vi "Drive Output Ramp.vi"(7 "reinitialize?":bool, 10 "Right":dbl, 11 "Left":dbl) -> (2 "Right Output":dbl, 3 "Left Output":dbl)   [LabVIEW 2013]
uses:
  <vilib>/addons/control/pid/pid.llb/PID Output Rate Limiter (DBL Array).vi
  <vilib>/addons/control/pid/NI_PID_pid.lvlib
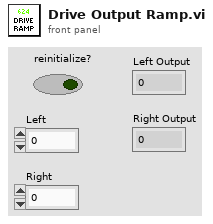
[diagram p1: front panel]
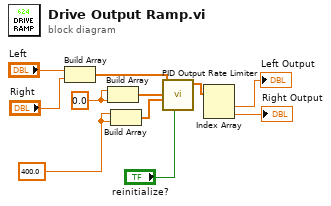
[diagram p0: block diagram]
diagram:
  w7 = 400.0 ("output rate (EGU/min)")
  w5 = 0.0 ("initial output")
  n1 = Build Array("Left", "Right") -> (w2:dbl[])
  n2 = Build Array(w5, w5) -> (w6:dbl[])
  n3 = Build Array(w7, w7) -> (w8:dbl[])
  n4 = call-poly <vilib>:"PID Output Rate Limiter.vi"("reinitialize? (F)"="reinitialize?", "output rate (EGU/min)"=w8, "initial output"=w6, "input (controller output)"=w2) -> ("output"=w9:dbl[])  [unwired: 4 in, 1 out]
  n5 = Index Array(array=w9) -> (element #1=→"Left Output":dbl, element #2=→"Right Output":dbl)  [unwired: 2 in]
